vi "TestExec.Test Metric Pareto.vi"(11 "Test History":T1) -> (2 "Counts":i32[](array[numeric]), 3 "Codes":i32[](array[numeric]))   [LabVIEW 2018]
uses:
  TestExec.Test Result Metric History.ctl
  Metrics/TestExec.Test Result Metric History Item.ctl
  <vilib>/KATE/SeqMgr/SeqMgr.Result State Enum.ctl
  <vilib>/KATE/SeqMgr/SeqMgr.lvlib
panel:
  # "Time                                           Test/UUT                      Result/Code                                 Description"
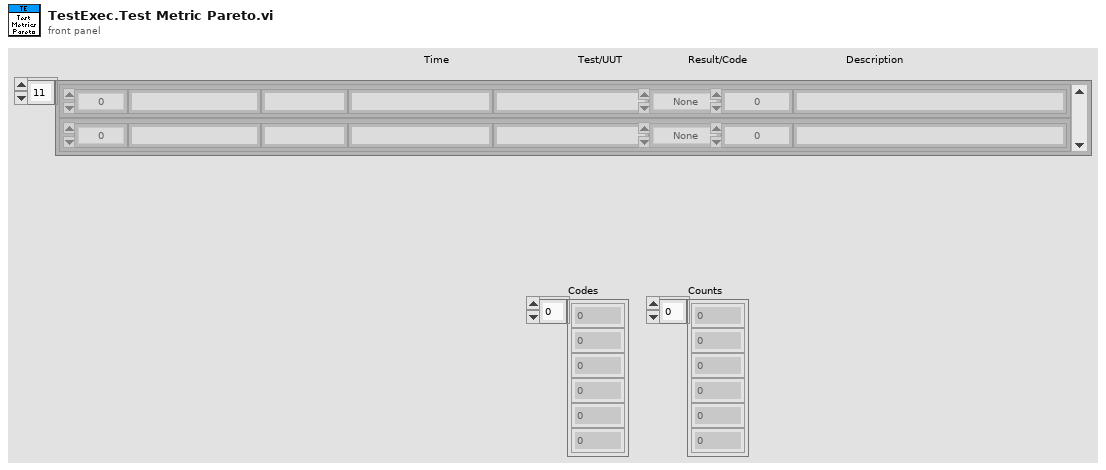
[diagram p1: front panel]
types:
  T1 = typedef "TestExec.Test Result Metric History.ctl" = T2[]
  T2 = typedef "TestExec.Test Result Metric History Item.ctl" = cluster{"TimeStamp":timestamp, "Dur(s)":dbl, "Time":string, "Mode ":string, "Test ":string, "SN":string, "State":T3, "Code":i32, "Description":string}
  T3 = typedef "KATE_Lib.lvlib/SeqMgr.lvlib/SeqMgr.Result State Enum.ctl" = enum16{"None", "Passing", "Failing", "PASS", "FAIL", "ABORT", "ERROR"}
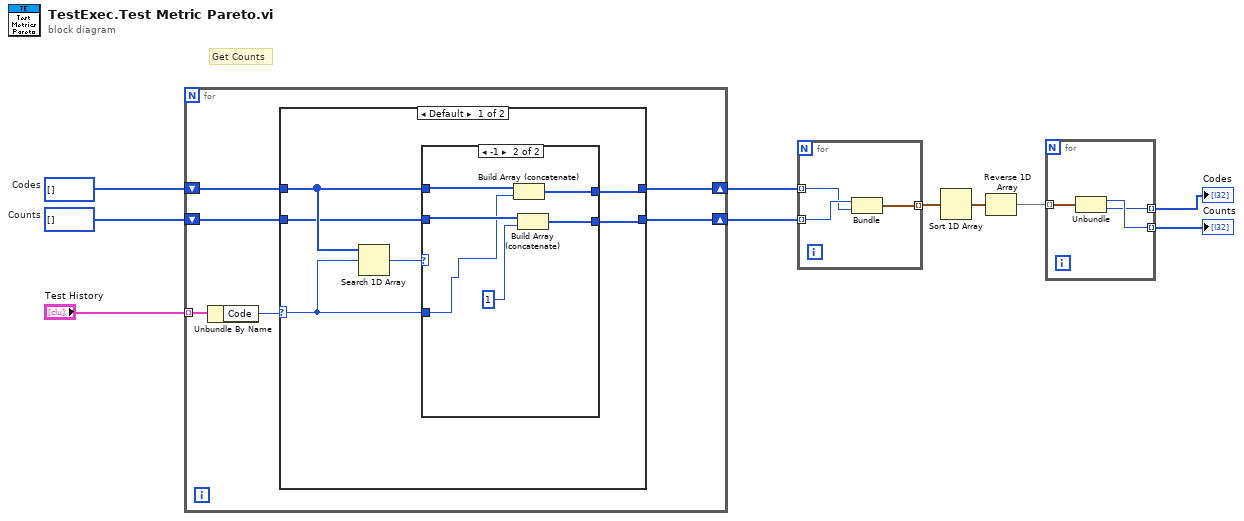
[diagram p0: block diagram]
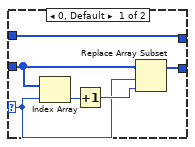
[diagram p2: hidden frame]
diagram:
  w9 = i32[] []  # Counts
  w8 = i32[] []  # Codes
  # "Get Counts"
  n1 = for {
    tunnel: "Test History" -> [w16] mode=indexing
    shift-right: [w11] -> w6
    shift-left: w9 -> [w12]
    shift-right: [w13] -> w7
    shift-left: w8 -> [w14]
    n2 = Unbundle By Name(w16) -> ("Code"=w15:i32)
    n3 = case shown="Default" w15 {
      selector: w15 -> [w17 _]
      tunnel: w14 -> [w21 w36]
      tunnel: [w19 w36] -> w13
      tunnel: w12 -> [w20 w35]
      tunnel: [w18 w35] -> w11
      frame Default {
        n4 = Search 1D Array(1D array=w21, element=w17) -> (index of element=w22:i32)  [unwired: 1 in]
        n5 = case shown="-1" w22 {
          selector: w22 -> [w23 _]
          tunnel: w21 -> [w28 w34]
          tunnel: w20 -> [w26 w32]
          tunnel: [w28 w33] -> w19
          tunnel: [w24 w30] -> w18
          tunnel: w17 -> [_ w29]
          frame 0, Default {
            n6 = Index Array(array=w26, index=w23) -> (element=w27:i32)
            n7 = Increment(x=w27) -> (x+1=w25:i32)
            n8 = Replace Array Subset(array=w26, new element=w25, index=w23) -> (w24:i32[])
          }
          frame -1 {
            n9 = Build Array (concatenate)(w34, w29) -> (w33:i32[])
            n10 = Build Array (concatenate)(w32, 1) -> (w30:i32[])
          }
        }
      }
      frame 0 {
      }
    }
  }
  n11 = for {
    tunnel: w7 -> [w38] mode=indexing
    tunnel: w6 -> [w39] mode=indexing
    tunnel: [w37] -> w5 mode=indexing
    n12 = Bundle(w39, w38) -> (w37:cluster{i32, i32})  [unwired: 1 in]
  }
  n13 = Sort 1D Array(array=w5) -> (sorted array=w2:cluster{i32, i32}[])
  n14 = Reverse 1D Array(array=w2) -> (reversed array=w1:cluster{i32, i32}[])
  n15 = for {
    tunnel: w1 -> [w42] mode=indexing
    tunnel: [w41] -> w4 mode=indexing
    tunnel: [w40] -> w3 mode=indexing
    n16 = Unbundle(w42) -> (w41:i32, w40:i32)
  }
  "Codes" <- w3
  "Counts" <- w4
